vi "CheckExt.vi"(1 "extension":string, 2 "Name in":string) -> (0 "Name":string)   [LabVIEW 2012]
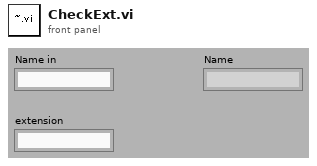
[diagram p1: front panel]
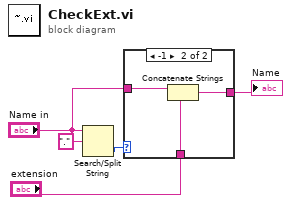
[diagram p0: block diagram]
diagram:
  n1 = Search/Split String(string="Name in", search string/char (-)=".") -> (offset of match=w2:i32)  [unwired: 1 in, 2 out]
  n2 = case shown="-1" w2 {
    tunnel: "Name in" -> [w6 w9]
    tunnel: [w6 w8] -> w4
    tunnel: "extension" -> [_ w7]
    frame Default {
    }
    frame -1 {
      n3 = Concatenate Strings(w9, w7) -> (w8:string)
    }
  }
  "Name" <- w4
